vi "Test Never Matching String Inputs Pass.vi"(8 "error in (no error)":errorcluster, 11 "Test Case In":refnum<class "Expectation Message Test.lvclass">) -> (0 "error out":errorcluster, 3 "Test Case Out":refnum<class "Expectation Message Test.lvclass">)   [LabVIEW 2020, in "Expectation Message Test.lvclass"]
uses:
  Expectation Message Test.lvclass
  C:/Program Files (x86)/National Instruments/LabVIEW 2020/vi.lib/Astemes/LUnit/Test Case.lvclass
  Test Doubles/Test Interface Responsive Mock/Test Interface Mock.lvclass
  C:/git/astemes-lmock/source/Framework/Mock/Mock.lvclass
  source/Expectations/Never/Never Matching String Inputs.vi
  source/Framework/LMock API.lvlib
  Expectation Test/Expectation Test.lvclass
  source/Expectations/Never/Never.lvlib
  C:/git/astemes-lmock/tests/Test Doubles/Test Interface Responsive Mock/Test Interface Mock.lvclass
  C:/git/astemes-lmock/tests/Test Doubles/Test Interface/Test Interface.lvclass
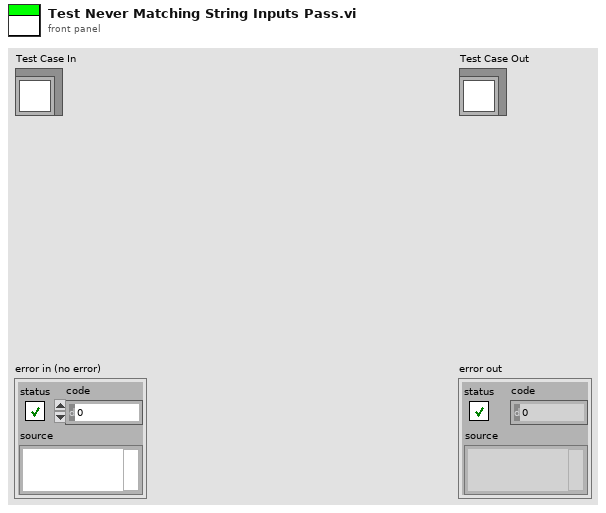
[diagram p1: front panel]
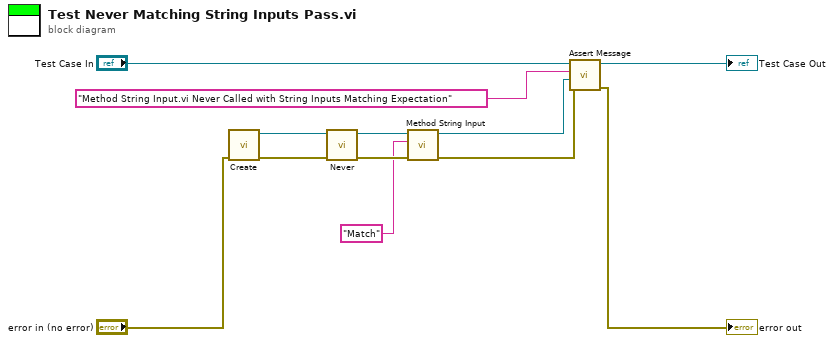
[diagram p0: block diagram]
diagram:
  n1 = call "Create.vi"("error in (no error)"="error in (no error)") -> ("error out"=w9:errorcluster, "Test Interface Mock Out"=w7:refnum<class "Test Interface Mock.lvclass">)  [unwired: 9 in]
  n2 = call-poly "Never.vi"("error in (no error)"=w9, "Mock in"=w7) -> ("error out"=w8:errorcluster, "Mock out"=w6:refnum<class "Test Interface Mock.lvclass">)  [unwired: 8 in]
  n3 = call-dynamic "Method String Input.vi"("error in (no error)"=w8, "String Input"="Match", "Test Interface Mock In"=w6) -> ("error out"=w3:errorcluster, "Test Interface Mock Out"=w2:refnum<class "Test Interface Mock.lvclass">)  [unwired: 7 in]
  n4 = call "Assert Message.vi"("error in (no error)"=w3, "Mock"=w2, "Message"="Method String Input.vi Never Called with String Inputs Matching Expectation", "LUnit Test Case In"="Test Case In") -> ("error out"=→"error out":errorcluster, "LUnit Test Case Out"=→"Test Case Out":refnum<class "Expectation Message Test.lvclass">)  [unwired: 6 in]
